vi "set_flexray_signal_raw_value.vi"(6 "AValue":dbl, 8 "error in (no error)":errorcluster caption="错误输入（无错误）", 9 "AData":u8, 10 "AFlexRaySignal":T1, 11 "path in":path) -> (0 "error out":errorcluster caption="错误输出", 2 "function return":i32, 3 "path out":path)   [LabVIEW 2014]
doc: "TSAPI(s32)set_flexray_signal_raw_value(const PMPFlexRaySignal AFlexRaySignal,const pu8 AData,const double AValue);"
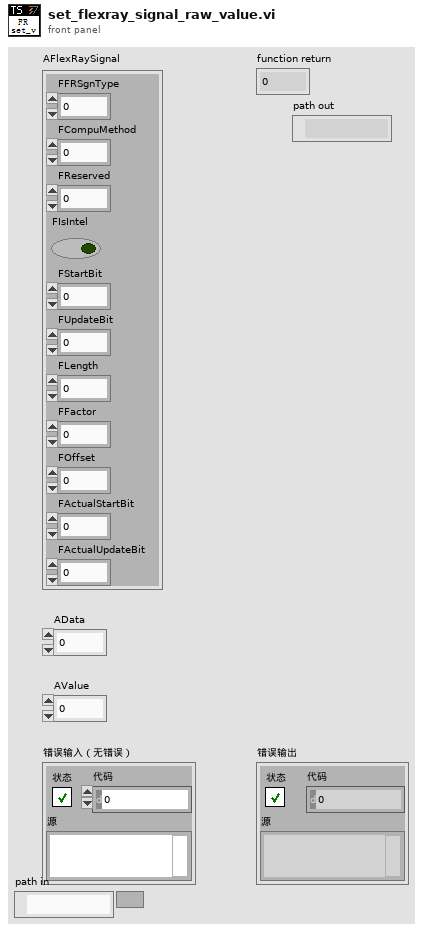
[diagram p1: front panel]
types:
  T1 = cluster{"FFRSgnType":u8, "FCompuMethod":u8, "FReserved":u8, "FIsIntel":bool, "FStartBit":i32, "FUpdateBit":i32, "FLength":i32, "FFactor":dbl, "FOffset":dbl, "FActualStartBit":i32, "FActualUpdateBit":i32}
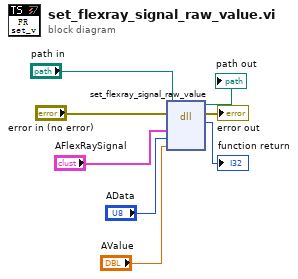
[diagram p0: block diagram]
diagram:
  n1 = dll-call lib="D:/Work/LabVIEW Code/TSMaster Labview SDK/LabVIEW/LabVIEW-TSMasterAPI_CLN/TSMasterAPI_LabVIEW-2024-10-08 14-20-13/Not_organized_vi/TSMaster.*" fn="set_flexray_signal_raw_value"(path in="path in", error in="error in (no error)", "AFlexRaySignal"="AFlexRaySignal", "AData"="AData", "AValue"="AValue") -> (path out=→"path out":path, error out=→"error out":errorcluster, "返回类型"=→"function return":i32)  [unwired: 4 in]
